vi "Build Class.vi"(7 "Actor Label":string, 8 "error in (no error)":errorcluster, 10 "Actor in":refnum<class "Engine.lvclass">, 11 "Engine in":refnum<class "Engine.lvclass">) -> (0 "error out":errorcluster, 2 "Actor out":refnum<class "Engine.lvclass">, 3 "Engine out":refnum<class "Engine.lvclass">)   [LabVIEW 2019, in "Engine.lvlib" / "Engine.lvclass"]
doc: "<b>Build Class</b>\nPre-populate the called class with universally accessible references/variables\n\n<b>Engine</b> Packs:\n Application Directory\n Event References\n Report Queue"
uses:
  Project/Engine.lvclass
  C:/Users/Public/Documents/Development/builds/Engine/Monitored Actor.lvlibp/Monitored Actor/Monitored Actor/Monitored Actor.lvclass
  Project/Engine.lvclass/Engine.ctl
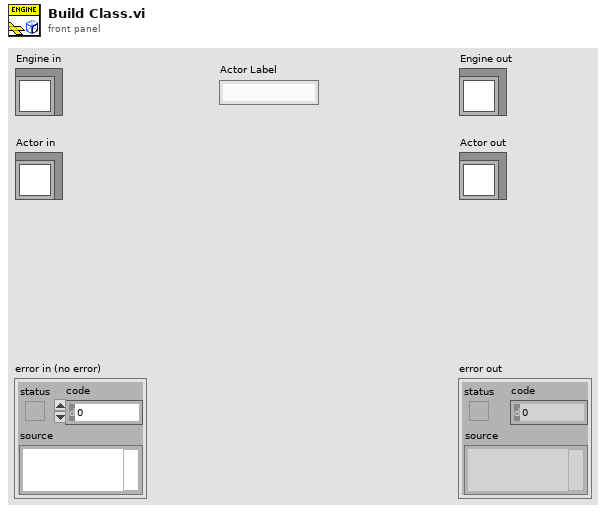
[diagram p1: front panel]
types:
  T1 = typedef "Engine.lvlib/Engine.lvclass/Engine Events.ctl" = cluster{"System Event":T2, "Manual":T3, "UUT":T4, "Interface Events":T5}
  T2 = typedef "Engine.lvlib/Engine.lvclass/System Events.ctl" = cluster{"Fault Event":refnum<user-event>, "SystemStatus Event":refnum<user-event>, "Automation":refnum<user-event>}
  T3 = typedef "Engine.lvlib/Engine.lvclass/Manual Events.ctl" = cluster{"QuickStart Event":refnum<user-event>, "SafeBTE Event":refnum<user-event>, "TogglePower Event":refnum<user-event>, "Change Instrument Event":refnum<user-event>, "Toggle Launch Event":refnum<user-event>, "UUTSupply":refnum<user-event>}
  T4 = typedef "Engine.lvlib/Engine.lvclass/UUT_Events.ctl" = cluster{"UUT_Name":refnum<user-event>, "Test_Name":refnum<user-event>, "Test_Operator":refnum<user-event>, "Test_Witness":refnum<user-event>, "Pedigree_Event":refnum<user-event>}
  T5 = typedef "Engine.lvlib/Engine.lvclass/Interface Events.ctl" = cluster{"Interface_Command":refnum<user-event>, "Telemetry_Descriptor":refnum<user-event>, "AsynchTLM_Descriptor":refnum<user-event>}
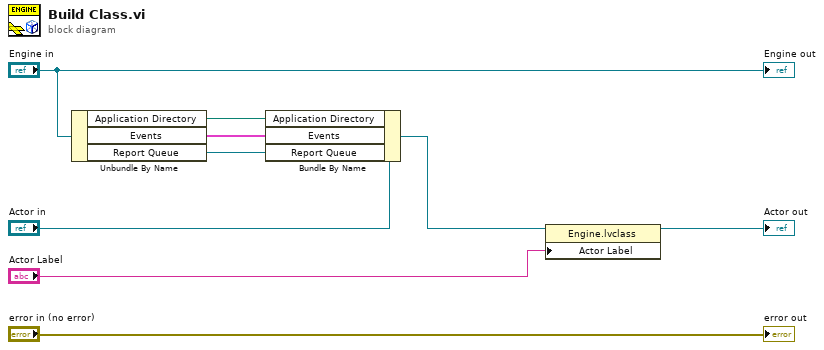
[diagram p0: block diagram]
diagram:
  n1 = Unbundle By Name("Engine in") -> ("Application Directory"=w6:path, "Events"=w4:T1, "Report Queue"=w3:refnum<class "QDMH.lvclass">)
  n2 = Bundle By Name(cluster="Actor in", "Application Directory"=w6, "Events"=w4, "Report Queue"=w3) -> (w7:refnum<class "Engine.lvclass">)
  n3 = property class="Engine.lvclass"(reference=w7, "Actor Label"="Actor Label") -> (reference out=→"Actor out":refnum<class "Engine.lvclass">)  [unwired: 1 in, 1 out]
  "error out" <- "error in (no error)"
  "Engine out" <- "Engine in"
